vi "Add Controls in Result.vi"(0 "VI Reference":refnum<vi>, 5 "Result Cluster":refnum<vi>, 7 "New Code Module":path, 11 "error in (no error)":errorcluster) -> (15 "error out":errorcluster)   [LabVIEW 2021, in "Converter.lvlib"]
uses:
  Converter.lvlib
  Converter Reusables/Converter Reusables.lvlib
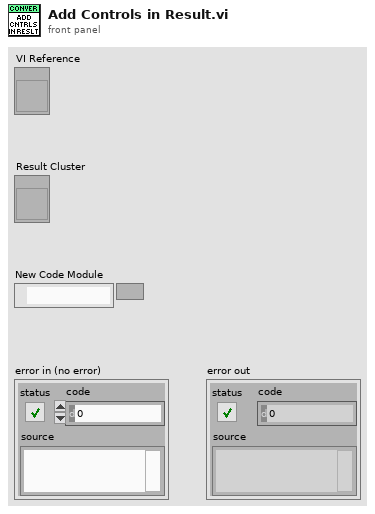
[diagram p1: front panel]
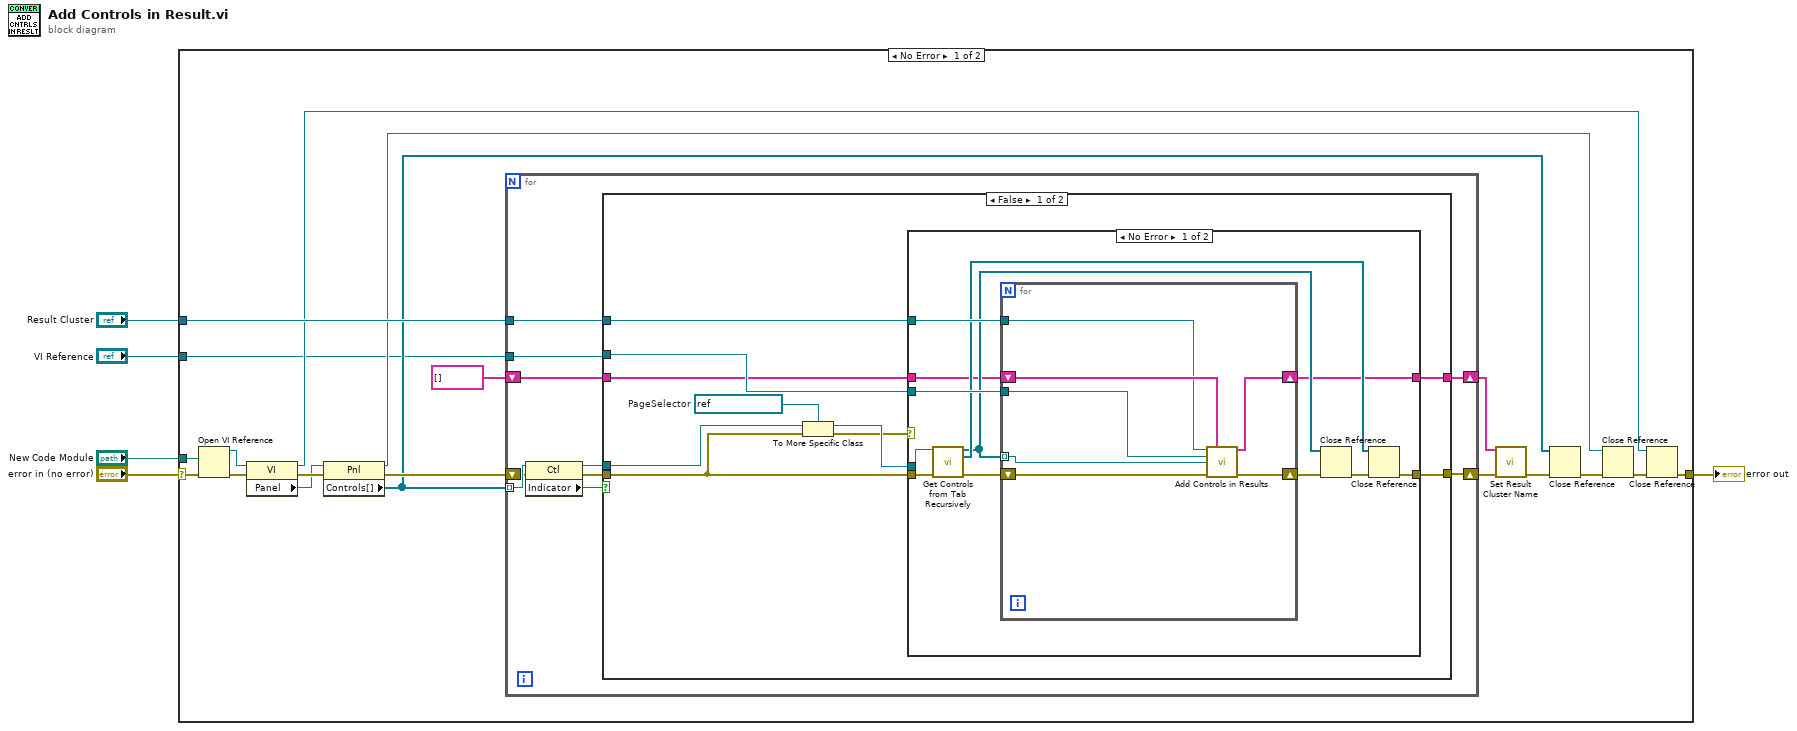
[diagram p0: block diagram]
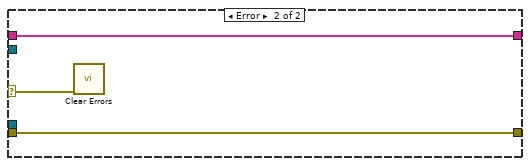
[diagram p2: hidden frame]
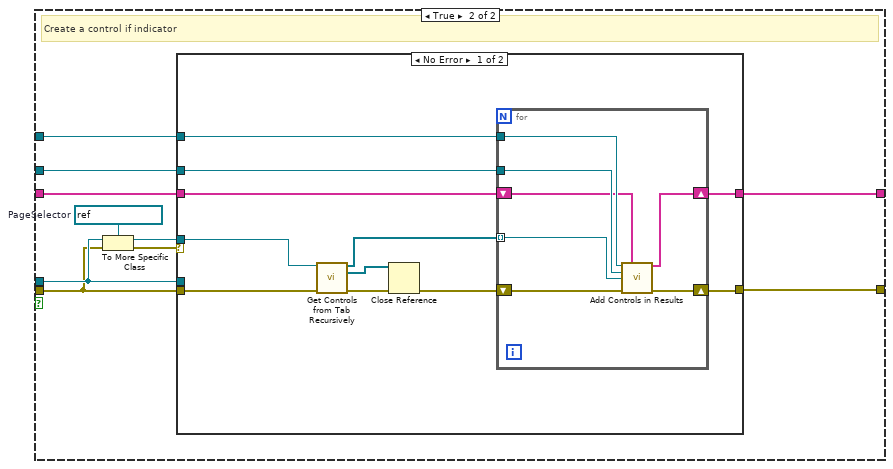
[diagram p3: hidden frame]
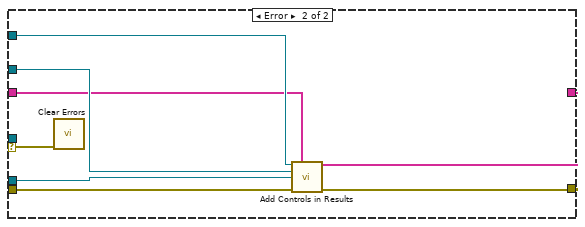
[diagram p4: hidden frame]
diagram:
  n1 = case shown="No Error" "error in (no error)" {
    selector: "error in (no error)" -> [w24 w103]
    tunnel: "New Code Module" -> [w23 _]
    tunnel: "Result Cluster" -> [w22 _]
    tunnel: [w14 w103] -> w2
    tunnel: "VI Reference" -> [w10 _]
    frame No Error {
      n2 = Open VI Reference(vi path=w23, error in (no error)=w24) -> (vi reference=w15:refnum<vi>, error out=w19:errorcluster)  [unwired: 4 in]
      n3 = property class="VI"(reference=w15, error in=w19) -> (reference out=w12:refnum<vi>, error out=w20:errorcluster, "Panel"=w17:refnum<vi>)
      n4 = property class="Pnl"(reference=w17, error in=w20) -> (reference out=w11:refnum<vi>, error out=w21:errorcluster, "Controls[]"=w18:refnum<vi>[])
      n5 = for {
        tunnel: w18 -> [w32] mode=indexing
        shift-right: [w33] -> w6
        shift-left: w21 -> [w30]
        tunnel: w22 -> [w34]
        tunnel: w10 -> [w27]
        shift-right: [w26] -> w8
        shift-left: string[] [] ("Output Clusters") -> [w25]
        n6 = property class="Ctl"(reference=w32, error in=w30) -> (reference out=w28:refnum<vi>, error out=w29:errorcluster, "Indicator"=w31:bool)
        n7 = case shown="False" w31 {
          tunnel: w34 -> [w37 w76]
          tunnel: w29 -> [w39 w72]
          tunnel: w28 -> [w44 w73]
          tunnel: [w41 w75] -> w33
          tunnel: w27 -> [w40 w74]
          tunnel: [w35 w68] -> w26
          tunnel: w25 -> [w36 w67]
          frame False {
            w43 = refnum<vi> refnum  # PageSelector
            n8 = To More Specific Class(target class=w43, reference=w44, error in=w39) -> (specific class reference=w42:refnum<vi>, error out=w38:errorcluster)
            n9 = case shown="No Error" w38 {
              selector: w38 -> [_ w66]
              tunnel: w42 -> [w56 _]
              tunnel: [w52 w65] -> w41
              tunnel: w40 -> [w51 _]
              tunnel: w39 -> [w50 w65]
              tunnel: w37 -> [w49 _]
              tunnel: w36 -> [w46 w64]
              tunnel: [w45 w64] -> w35
              frame No Error {
                n10 = call "Get Controls from Tab Recursively.vi"("PageSel Refnum"=w56, "error in (no error)"=w50) -> ("Indicators in Tab"=w47:refnum<vi>[], "Controls in Tab"=w48:refnum<vi>[], "error out"=w55:errorcluster)  [unwired: 11 in]
                n11 = for {
                  shift-right: [w58] -> w54
                  shift-left: w55 -> [w57]
                  tunnel: w47 -> [w59] mode=indexing
                  tunnel: w51 -> [w60]
                  tunnel: w49 -> [w61]
                  shift-right: [w62] -> w45
                  shift-left: w46 -> [w63]
                  n12 = call "Add Controls in Results.vi"("Result Cluster"=w61, "Output Clusters in"=w63, "VI Reference"=w60, "Ctl Refnum"=w59, "error in"=w57) -> ("Output Clusters out"=w62:string[], "error out"=w58:errorcluster)  [unwired: 9 in]
                }
                n13 = Close Reference(reference=w47, error in (no error)=w54) -> (error out=w53:errorcluster)
                n14 = Close Reference(reference=w48, error in (no error)=w53) -> (error out=w52:errorcluster)
              }
              frame Error {
                n15 = call <vilib>:"Clear Errors.vi"("error in (no error)"=w66) -> ()  [unwired: 5 in, 2 out]
              }
            }
          }
          frame True {
            w71 = refnum<vi> refnum  # PageSelector
            # "Create a control if indicator"
            n16 = To More Specific Class(target class=w71, reference=w73, error in=w72) -> (specific class reference=w69:refnum<vi>, error out=w70:errorcluster)
            n17 = case shown="No Error" w70 {
              selector: w70 -> [_ w99]
              tunnel: w76 -> [w81 w102]
              tunnel: [w79 w101] -> w75
              tunnel: w74 -> [w80 w100]
              tunnel: w73 -> [_ w98]
              tunnel: w72 -> [w86 w95]
              tunnel: w69 -> [w87 _]
              tunnel: [w77 w97] -> w68
              tunnel: w67 -> [w78 w96]
              frame No Error {
                n18 = call "Get Controls from Tab Recursively.vi"("PageSel Refnum"=w87, "error in (no error)"=w86) -> ("Indicators in Tab"=w83:refnum<vi>[], "Controls in Tab"=w85:refnum<vi>[], "error out"=w84:errorcluster)  [unwired: 11 in]
                n19 = Close Reference(reference=w85, error in (no error)=w84) -> (error out=w82:errorcluster)
                n20 = for {
                  tunnel: w83 -> [w91] mode=indexing
                  tunnel: w81 -> [w93]
                  shift-right: [w90] -> w79
                  shift-left: w82 -> [w94]
                  tunnel: w80 -> [w92]
                  shift-right: [w88] -> w77
                  shift-left: w78 -> [w89]
                  n21 = call "Add Controls in Results.vi"("Result Cluster"=w93, "Output Clusters in"=w89, "VI Reference"=w92, "Ctl Refnum"=w91, "error in"=w94) -> ("Output Clusters out"=w88:string[], "error out"=w90:errorcluster)  [unwired: 9 in]
                }
              }
              frame Error {
                n22 = call <vilib>:"Clear Errors.vi"("error in (no error)"=w99) -> ()  [unwired: 5 in, 2 out]
                n23 = call "Add Controls in Results.vi"("Result Cluster"=w102, "Output Clusters in"=w96, "VI Reference"=w100, "Ctl Refnum"=w98, "error in"=w95) -> ("Output Clusters out"=w97:string[], "error out"=w101:errorcluster)  [unwired: 9 in]
              }
            }
          }
        }
      }
      n24 = call "Set Result Cluster Name.vi"("Controls Name"=w8, "error in (no error)"=w6) -> ("error out"=w7:errorcluster)  [unwired: 13 in]
      n25 = Close Reference(reference=w18, error in (no error)=w7) -> (error out=w16:errorcluster)
      n26 = Close Reference(reference=w11, error in (no error)=w16) -> (error out=w13:errorcluster)
      n27 = Close Reference(reference=w12, error in (no error)=w13) -> (error out=w14:errorcluster)
    }
    frame Error {
    }
  }
  "error out" <- w2
